vi "Proto Key And Type.vi"(11 "Array":u8[](array[numeric]) format="%02x") -> (1 "array w/ subset deleted":u8[](array[numeric]), 2 "Key":i32, 3 "Type":i32)   [LabVIEW 2018]
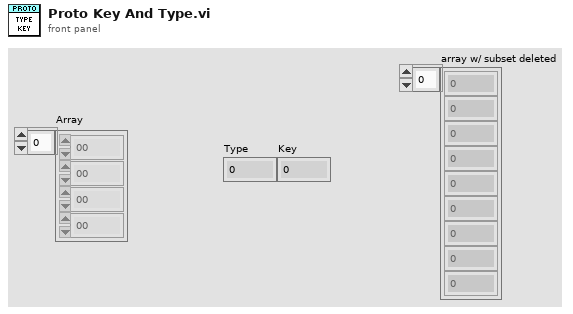
[diagram p1: front panel]
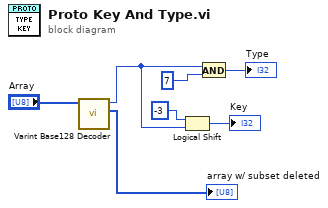
[diagram p0: block diagram]
diagram:
  n1 = call "Varint Base128 Decoder.vi"("Array"="Array") -> ("array w/ subset deleted"=→"array w/ subset deleted":u8[], "Numeric"=w4:i32)  [unwired: 9 in]
  n2 = Logical Shift(y=i16 -3, x=w4) -> (x << y=→"Key":i32)
  n3 = And(x=w4, y=7) -> (x .and. y?=→"Type":i32)
